vi "RUSHBridge.vi"(7 "Up to Down":bool, 9 "RA Down Volt":dbl, 10 "RA Up Volt":dbl, 11 "Voltage":dbl) -> (2 "Ramp Actuator Ouput":dbl)   [LabVIEW 2011]
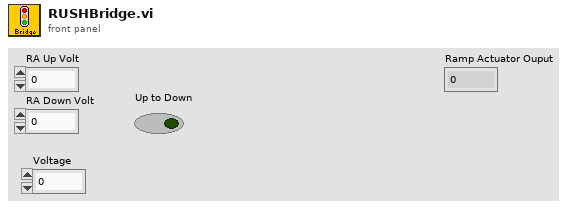
[diagram p1: front panel]
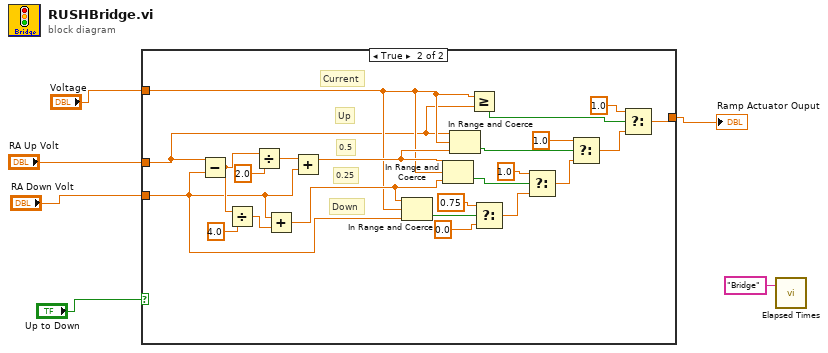
[diagram p0: block diagram]
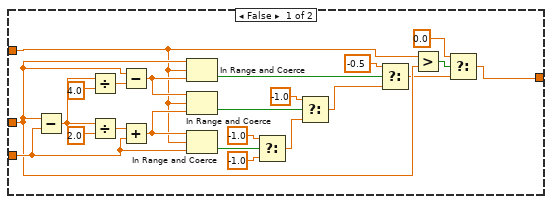
[diagram p2: hidden frame]
diagram:
  n1 = case shown="True" "Up to Down" {
    tunnel: "RA Down Volt" -> [w24 w36]
    tunnel: "Voltage" -> [w7 w35]
    tunnel: "RA Up Volt" -> [w12 w34]
    tunnel: [w8 w30] -> w3
    frame False {
      n2 = Subtract(x=w12, y=w24) -> (x-y=w27:dbl)
      n3 = Divide(x=w27, y=4.0) -> (x/y=w25:dbl)
      n4 = Divide(x=w27, y=2.0) -> (x/y=w28:dbl)
      n5 = Subtract(x=w12, y=w25) -> (x-y=w14:dbl)
      n6 = Add(x=w28, y=w24) -> (x+y=w16:dbl)
      n7 = In Range and Coerce(upper limit=w12, x=w7, lower limit=w14) -> (In Range?=w13:bool)  [unwired: 1 out]
      n8 = In Range and Coerce(upper limit=w14, x=w7, lower limit=w16) -> (In Range?=w15:bool)  [unwired: 1 out]
      n9 = In Range and Coerce(upper limit=w16, x=w7, lower limit=w24) -> (In Range?=w23:bool)  [unwired: 1 out]
      n10 = Select(t=-1.0, s=w23, f=-1.0) -> (s? t:f=w20:dbl)
      n11 = Select(t=-1.0, s=w15, f=w20) -> (s? t:f=w18:dbl)
      n12 = Select(t=-0.5, s=w13, f=w18) -> (s? t:f=w11:dbl)
      n13 = Greater?(x=w7, y=w12) -> (0:w10:bool)
      n14 = Select(t=0.0, s=w10, f=w11) -> (s? t:f=w8:dbl)
    }
    frame True {
      # "Current"
      # "Down"
      # "0.25"
      # "0.5"
      # "Up"
      n15 = Subtract(x=w34, y=w36) -> (x-y=w49:dbl)
      n16 = Divide(x=w49, y=4.0) -> (x/y=w48:dbl)
      n17 = Divide(x=w49, y=2.0) -> (x/y=w50:dbl)
      n18 = Add(x=w36, y=w48) -> (x+y=w38:dbl)
      n19 = Add(x=w50, y=w36) -> (x+y=w37:dbl)
      n20 = In Range and Coerce(upper limit=w38, x=w35, lower limit=w36) -> (In Range?=w40:bool)  [unwired: 1 out]
      n21 = In Range and Coerce(upper limit=w37, x=w35, lower limit=w38) -> (In Range?=w44:bool)  [unwired: 1 out]
      n22 = In Range and Coerce(upper limit=w34, x=w35, lower limit=w37) -> (In Range?=w39:bool)  [unwired: 1 out]
      n23 = Greater Or Equal?(x=w35, y=w34) -> (x >= y?=w33:bool)
      n24 = Select(t=0.75, s=w40, f=0.0) -> (s? t:f=w43:dbl)
      n25 = Select(t=1.0, s=w44, f=w43) -> (s? t:f=w46:dbl)
      n26 = Select(t=1.0, s=w39, f=w46) -> (s? t:f=w31:dbl)
      n27 = Select(t=1.0, s=w33, f=w31) -> (s? t:f=w30:dbl)
    }
  }
  "Ramp Actuator Ouput" <- w3
  n28 = call "Elapsed Times.vi"("Call Name"="Bridge") -> ()  [unwired: 2 in, 1 out]
